vi "measure_NI.vi"(1 "XY-in":dbl[](array[numeric]), 2 "bar-note":u8, 7 "stage-refs":T2, 11 "stage-error-in":errorcluster, 12 "counter-in":dbl format="%#_13g", 13 "meas#":dbl) -> (3 "measured-point out":dbl[](array[numeric]), 4 "logfile-line-out":string, 6 "iCorr-out":dbl, 8 "PD out":T1, 14 "counter-out":dbl, 15 "stage-error-out":errorcluster)   [LabVIEW 2024]
uses:
  C:/Users/hpDIRC/Desktop/eic_dirc_daq-LabVIEW_new/Thorlabs/Thorlabs.MotionControl.IntegratedStepperMotorsCLI.dll
  Thorlabs/Thorlabs.MotionControl.IntegratedStepperMotorsCLI.dll
  C:/Users/hpDIRC/Desktop/eic_dirc_daq-LabVIEW_new/Thorlabs/Thorlabs.MotionControl.Benchtop.StepperMotorCLI.dll
  Thorlabs/Thorlabs.MotionControl.Benchtop.StepperMotorCLI.dll
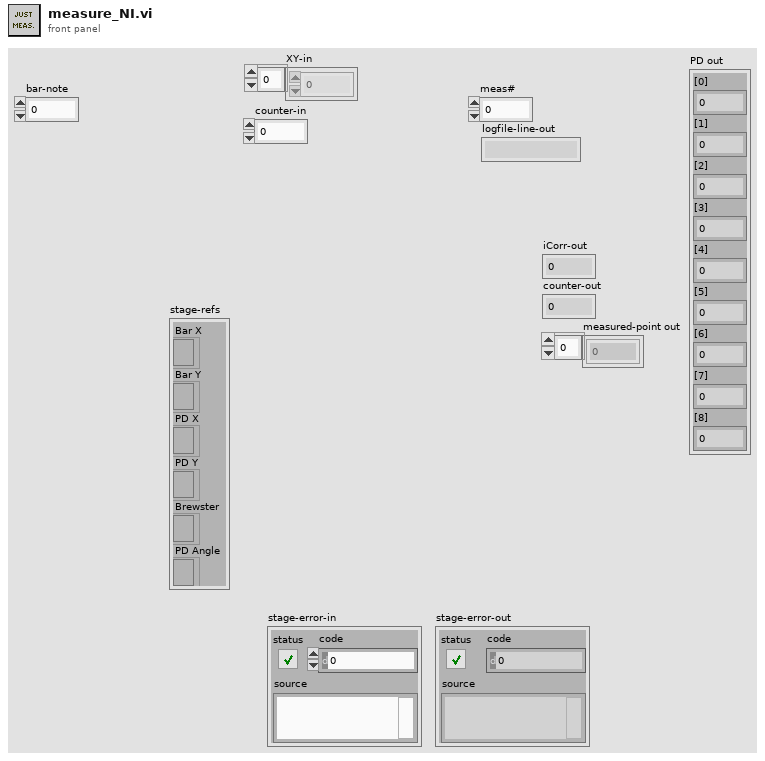
[diagram p1: front panel]
types:
  T1 = cluster{"[0]":dbl, "[1]":dbl, "[2]":dbl, "[3]":dbl, "[4]":dbl, "[5]":dbl, "[6]":dbl, "[7]":dbl, "[8]":dbl}
  T2 = cluster{"Bar X":refnum<k24>, "Bar Y":refnum<k24>, "PD X":refnum<k24>, "PD Y":refnum<k24>, "Brewster":refnum<k24>, "PD Angle":refnum<k24>}
  T3 = cluster{"Bar X":dbl, "Bar Y":dbl, "PD X":dbl, "PD Y":dbl, "BMA":dbl, "PDA":dbl}
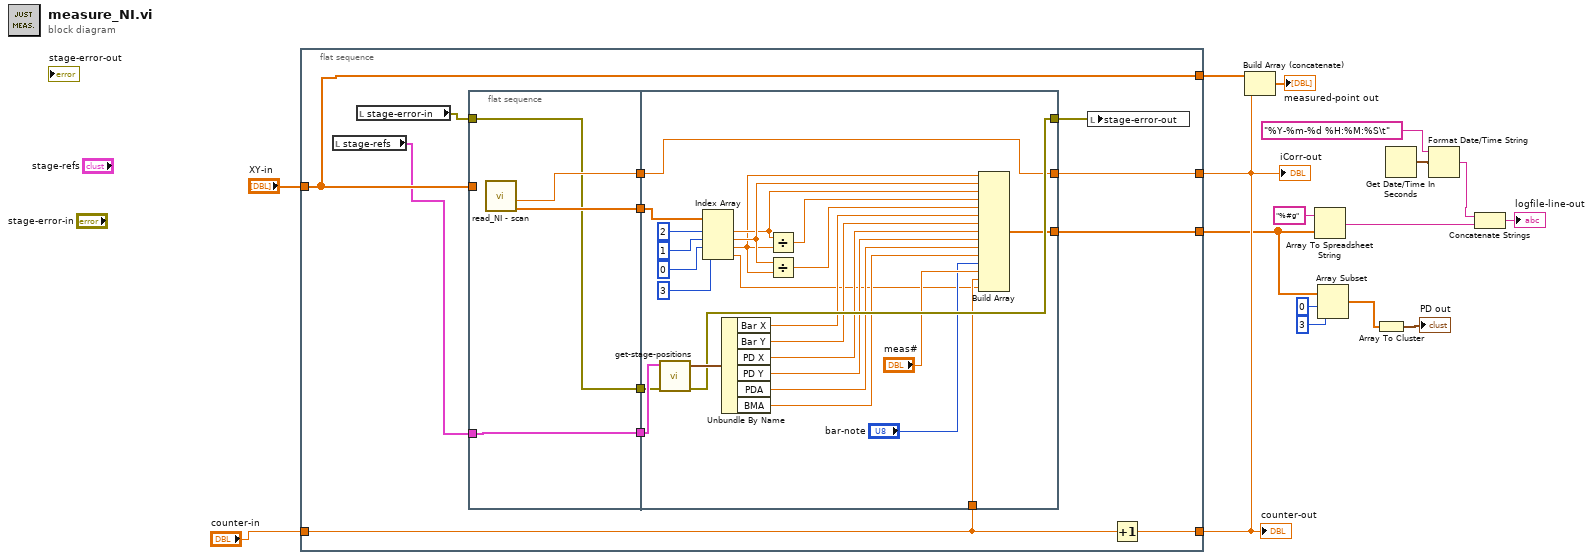
[diagram p0: block diagram]
diagram:
  n1 = flat-sequence {
    tunnel: [w29] -> w13
    tunnel: "XY-in" -> [w26]
    tunnel: "counter-in" -> [w19]
    tunnel: [w20] -> w12
    tunnel: [w26] -> w14
    tunnel: [w18] -> w5
    frame #0 {
      n2 = local read "stage-refs"() -> (w22:T2)
      n3 = local read "stage-error-in"() -> (w27:errorcluster)
      n4 = flat-sequence {
        tunnel: [w31] -> w25
        tunnel: [w32] -> w24
        tunnel: [w33] -> w23
        tunnel: [w30] -> w21
        tunnel: w27 -> [w30]
        tunnel: w26 -> [_]
        tunnel: w22 -> [w33]
        tunnel: [w50] -> w28
        tunnel: [w39] -> w29
        tunnel: w25 -> [w39]
        tunnel: w24 -> [w56]
        tunnel: w23 -> [w52]
        tunnel: w21 -> [w51]
        tunnel: w19 -> [w43]
        tunnel: [w41] -> w18
        frame #0 {
          n5 = call "read_NI - scan.vi"() -> ("all_pds"=w32:dbl[], "-pd3/pd1"=w31:dbl)  [unwired: 8 in, 2 out]
        }
        frame #1 {
          n6 = call "get-stage-positions.vi"("error in (no error)"=w51, "Cluster"=w52) -> ("error out"=w50:errorcluster, "stage positions"=w53:T3)  [unwired: 8 in]
          n7 = Index Array(array=w56, index #1=2 ("index"), index #2=1 ("index"), index #3=0 ("index"), index #4=3 ("index")) -> (element #1=w38:dbl, element #2=w40:dbl, element #3=w36:dbl, element #4=w34:dbl)
          n8 = Unbundle By Name(w53) -> ("Bar X"=w49:dbl, "Bar Y"=w48:dbl, "PD X"=w47:dbl, "PD Y"=w46:dbl, "PDA"=w45:dbl, "BMA"=w44:dbl)
          n9 = Divide(x=w38, y=w36) -> (x/y=w55:dbl)
          n10 = Divide(x=w40, y=w36) -> (x/y=w54:dbl)
          n11 = Build Array(w36, w40, w38, w55, w54, w49, w48, w47, w46, w45, w44, "bar-note", "meas#", w43, w34) -> (w41:dbl[])
        }
      }
      n12 = local write "stage-error-out"(w28) -> ()
      n13 = Increment(x=w19) -> (x+1=w20:dbl)
    }
  }
  n14 = Build Array (concatenate)(w14, w13, w12) -> (→"measured-point out":dbl[])
  n15 = Array To Spreadsheet String(array=w5, 3:"%#g" ("format string")) -> (spreadsheet string=w8:string)  [unwired: 1 in]
  n16 = Array Subset(array=w5, index=0, length=3) -> (w2:dbl[])
  n17 = Array To Cluster(array=w2) -> (cluster=→"PD out":T1)
  n18 = Get Date/Time In Seconds() -> (seconds since 1Jan1904=w11:timestamp)
  n19 = Format Date/Time String(time format string (%c)="%Y-%m-%d %H:%M:%S\t", seconds (now)=w11) -> (date/time string=w7:string)  [unwired: 1 in]
  n20 = Concatenate Strings(w7, w8) -> (→"logfile-line-out":string)
  "iCorr-out" <- w13
  "counter-out" <- w12
